vi "iHR550 Init.vi"(1 "Mono ID":refnum<vi>, 2 "Target ID":string="iHR550") -> ()   [LabVIEW 2010]
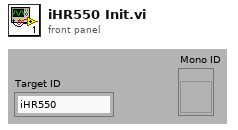
[diagram p1: front panel]
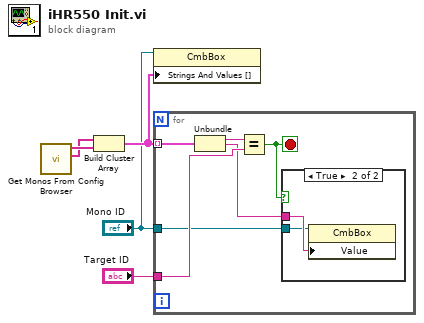
[diagram p0: block diagram]
diagram:
  n1 = call "Get Monos From Config Browser.vi"() -> ("UniqueIDs"=w5:string[], "Mono ID"=w4:string[])  [unwired: 3 in, 1 out]
  n2 = Build Cluster Array(w4, w5) -> (w3:cluster{"String":string, "String":string}[])
  n3 = property on="Eigenschaftsknoten" class="CmbBox"(reference="Mono ID", "Strings And Values []"=w3) -> ()  [unwired: 1 in, 2 out]
  n4 = for {
    tunnel: w3 -> [w11] mode=indexing
    tunnel: "Target ID" -> [w9]
    tunnel: "Mono ID" -> [w6]
    stop <- w8 stop-if-true
    n5 = Unbundle(w11) -> ("String"=w10:string, "String"=w7:string)
    n6 = Equal?(x=w10, y=w9) -> (x = y?=w8:bool)
    n7 = case shown="True" w8 {
      tunnel: w7 -> [_ w13]
      tunnel: w6 -> [_ w12]
      frame False {
      }
      frame True {
        n8 = property class="CmbBox"(reference=w12, "Value"=w13) -> ()  [unwired: 1 in, 2 out]
      }
    }
  }
